vi "svl_Log View for Energy Level (N Ch) (array).vi"(8 "error in (no error)":errorcluster, 9 "view mode":enum16{"Power", "Amplitude"}(ring), 10 "dB On (T)":bool=TRUE, 11 "scaled signals":waveform(dbl)[](array[waveform])) -> (0 "error out":errorcluster, 1 "unit labels":string[](array[string]), 3 "scaled signals":waveform(dbl)[](array[waveform]))   [LabVIEW 2017]
uses:
  <vilib>/addons/_NISVFA/_Shared subVIs/Common/svc_Engineering Units to Unit Label.vi
  <vilib>/addons/_NISVFA/_Shared subVIs/Common/svc_Unit Label to Engineering Units.vi
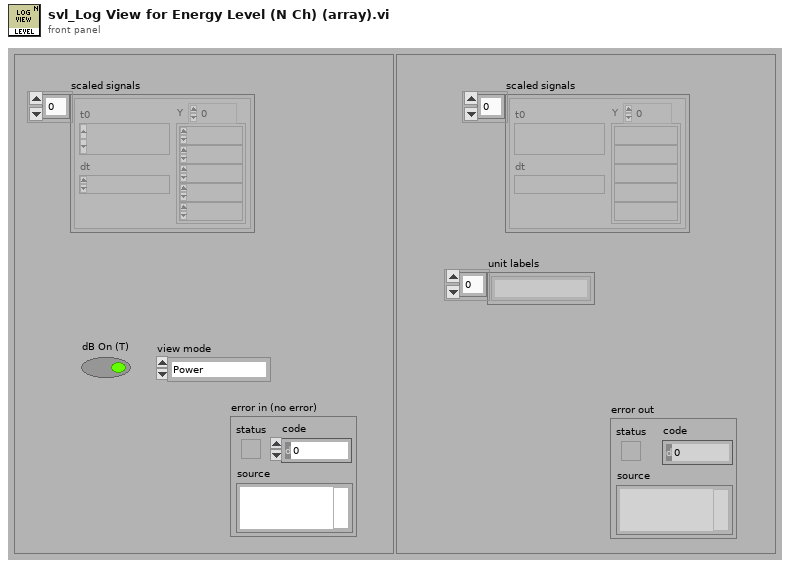
[diagram p1: front panel]
types:
  T1 = typedef "svc_Channel Info.ctl" = cluster{"sensor sensitivity":dbl, "engineering units":T2, "dB reference":dbl, "custom label":string, "weighting filter":T3, "pregain":dbl}
  T2 = typedef "svc_Engineering Units Text Ring.ctl" = u16
  T3 = typedef "svc_Weighting Filter Text Ring.ctl" = u16
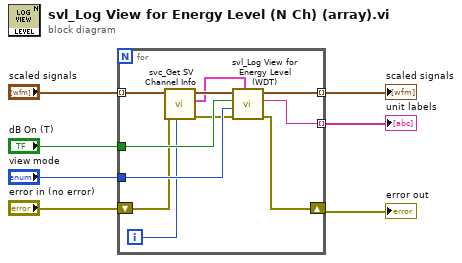
[diagram p0: block diagram]
diagram:
  n1 = for {
    tunnel: "scaled signals" -> [w10] mode=indexing
    tunnel: [w17] -> w6 mode=indexing
    tunnel: [w14] -> w7 mode=indexing
    tunnel: "view mode" -> [w16]
    tunnel: "dB On (T)" -> [w15]
    shift-right: [w18] -> w4
    shift-left: "error in (no error)" -> [w13]
    i -> [w8]
    n2 = call <vilib>:"svc_Get SV Channel Info.vi"("channel index"=w8, "error in (no error)"=w13, "scaled signal [EU]"=w10) -> ("error out"=w12:errorcluster, "channel info"=w9:T1, "dup scaled signal [EU]"=w11:waveform(dbl))  [unwired: 3 in, 3 out]
    n3 = call <vilib>:"svl_Log View for Energy Level (WDT).vi"("channel info"=w9, "error in (no error)"=w12, "view mode"=w16, "dB On (T)"=w15, "scaledSignal"=w11) -> ("error out"=w18:errorcluster, "unit label"=w17:string, "scaledSignal"=w14:waveform(dbl))  [unwired: 4 in]
  }
  "scaled signals" <- w7
  "unit labels" <- w6
  "error out" <- w4
